vi "changestring.vi"() -> ()   [LabVIEW 2022 SP3]
panel:
  in  "停止":bool
  in  "字符串":string="ABC"
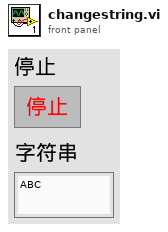
[diagram p1: front panel]
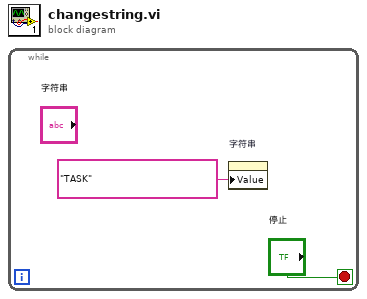
[diagram p0: block diagram]
diagram:
  n1 = while {
    stop <- "停止" stop-if-true
    n2 = property on="字符串" class="Str"("Value"="TASK") -> ()  [unwired: 2 in, 2 out]
  }
